vi "DT_Triangle Manager_Get Global Point Index.vi"(9 "local idx":i32, 10 "triangle":i32, 11 "Triangles":i32[][](array[numeric])) -> (2 "global idx":i32)   [LabVIEW 2017, in "NI_AAL_Geometry.lvlib"]
uses:
  <vilib>/Analysis/NI_AAL_Geometry.lvlib
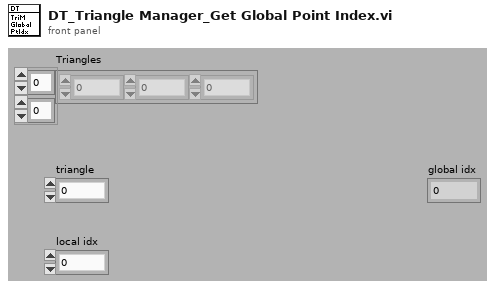
[diagram p1: front panel]
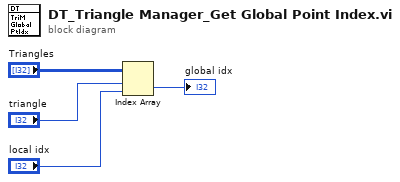
[diagram p0: block diagram]
diagram:
  n1 = Index Array(array="Triangles", index (row)="triangle", index (col)="local idx") -> (element=→"global idx":i32)
